vi "FlatToRichnixnet_grpc_FlexRayStats.vi"(5 "OutputClusterType":T1, 11 "InputCluster":T2) -> (3 "OutputCluster":T1)   [LabVIEW 2025, in "xnet-grpc_client.lvlib"]
uses:
  xnet-grpc_client.lvlib
  nixnet_grpc_FlexRayStats_Flat.ctl
  nixnet_grpc_FlexRayStats.ctl
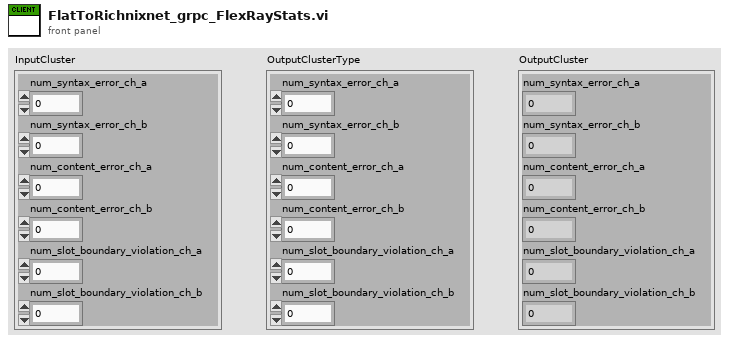
[diagram p1: front panel]
types:
  T1 = typedef "xnet-grpc_client.lvlib/nixnet_grpc_FlexRayStats.ctl" = cluster{"num_syntax_error_ch_a":u32, "num_syntax_error_ch_b":u32, "num_content_error_ch_a":u32, "num_content_error_ch_b":u32, "num_slot_boundary_violation_ch_a":u32, "num_slot_boundary_violation_ch_b":u32}
  T2 = typedef "xnet-grpc_client.lvlib/nixnet_grpc_FlexRayStats_Flat.ctl" = cluster{"num_syntax_error_ch_a":u32, "num_syntax_error_ch_b":u32, "num_content_error_ch_a":u32, "num_content_error_ch_b":u32, "num_slot_boundary_violation_ch_a":u32, "num_slot_boundary_violation_ch_b":u32}
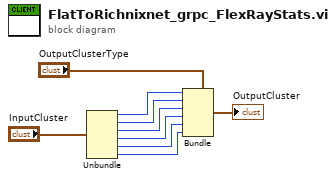
[diagram p0: block diagram]
diagram:
  n1 = Unbundle "Unbundle"("InputCluster") -> ("num_syntax_error_ch_a"=w6:u32, "num_syntax_error_ch_b"=w5:u32, "num_content_error_ch_a"=w4:u32, "num_content_error_ch_b"=w3:u32, "num_slot_boundary_violation_ch_a"=w2:u32, "num_slot_boundary_violation_ch_b"=w1:u32)
  n2 = Bundle "Bundle"(cluster="OutputClusterType", "num_syntax_error_ch_a"=w6, "num_syntax_error_ch_b"=w5, "num_content_error_ch_a"=w4, "num_content_error_ch_b"=w3, "num_slot_boundary_violation_ch_a"=w2, "num_slot_boundary_violation_ch_b"=w1) -> (→"OutputCluster":T1)
